vi "read_sudoku.vi"(11 "path to JPEG file":path) -> (0 "gestion des erreurs":errorcluster, 1 "image data":T1, 2 "image data 2":T1, 3 "new picture":picture, 4 "Rectangle.right":i16, 5 "Rectangle.bottom":i16)   [LabVIEW 2023]
uses:
  <vilib>/picture/picture.llb/imagedata.ctl
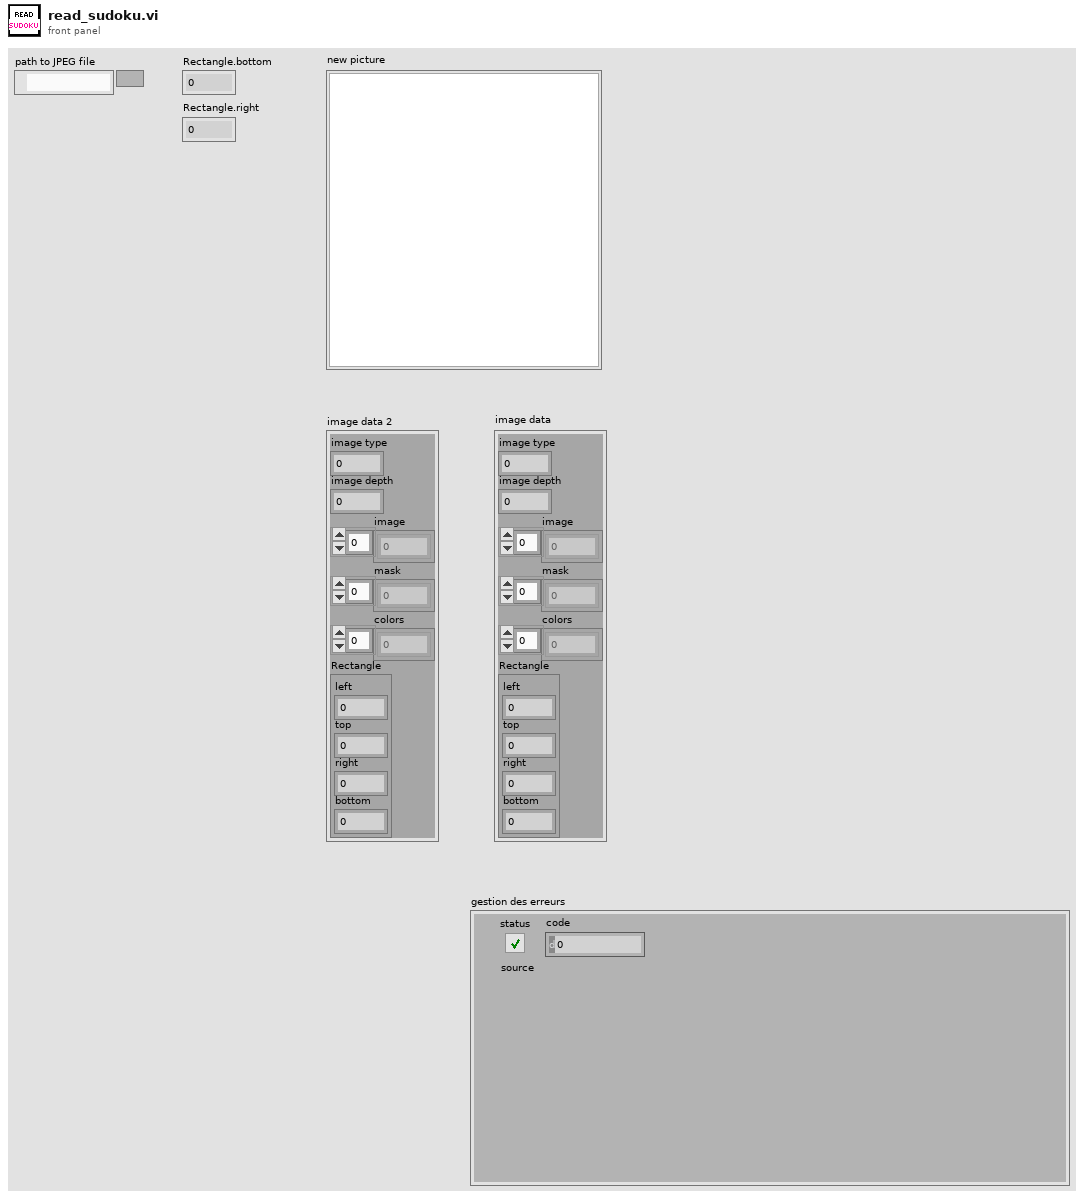
[diagram p1: front panel]
types:
  T1 = typedef "imagedata.ctl" = cluster{"image type":i32, "image depth":i32, "image":u8[], "mask":u8[], "colors":u32[], "Rectangle":cluster{"left":i16, "top":i16, "right":i16, "bottom":i16}}
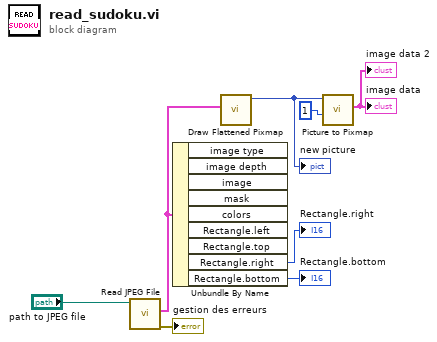
[diagram p0: block diagram]
diagram:
  n1 = call <vilib>:"Read JPEG File.vi"("path to JPEG file"="path to JPEG file") -> ("error out"=→"gestion des erreurs":errorcluster, "image data"=w3:T1)  [unwired: 8 in, 1 out]
  n2 = Unbundle By Name(w3) -> ("Rectangle.right"=→"Rectangle.right":i16, "Rectangle.bottom"=→"Rectangle.bottom":i16)  [unwired: 7 out]
  n3 = call <vilib>:"Draw Flattened Pixmap.vi"("image data"=w3) -> ("new picture"=w2:picture)  [unwired: 8 in]
  "new picture" <- w2
  n4 = call <vilib>:"Picture to Pixmap.vi"("depth"=1, "picture"=w2) -> ("image data"=→"image data" →"image data 2":T1)  [unwired: 8 in, 1 out]
